vi "RoiSelectionCoordinatesAndorNull_FGV.vi"(8 "error in":errorcluster, 10 "FGV_Control":enum16{"Set", "Get"}(ring), 11 "ROI Coordinates in":T1) -> (0 "error out":errorcluster, 3 "ROI Coordinates out":T1)   [LabVIEW 2010]
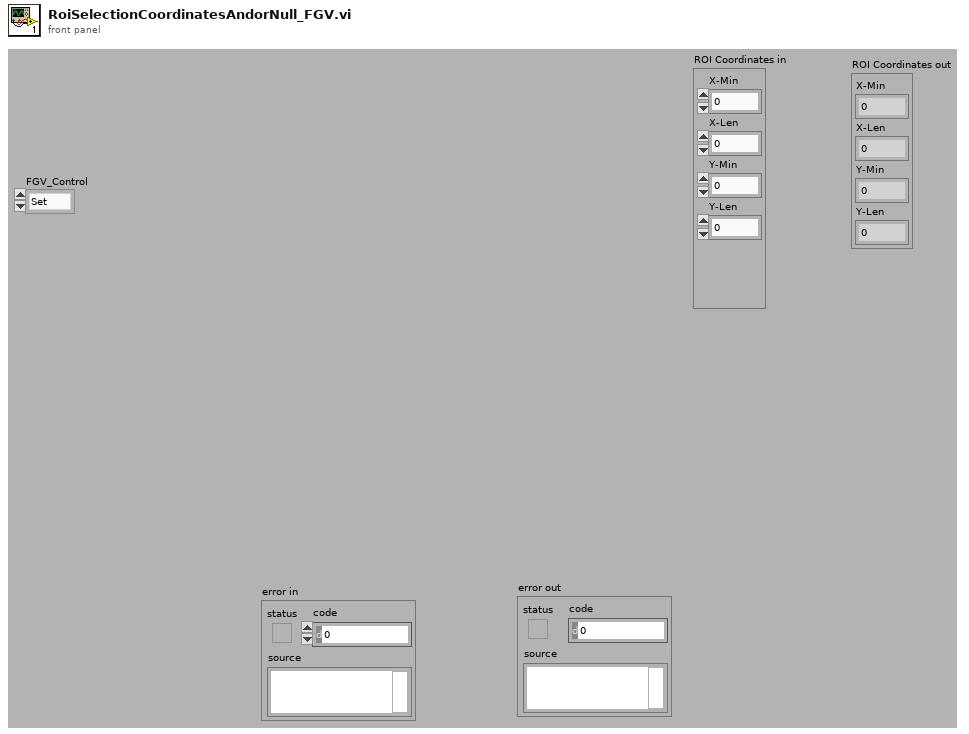
[diagram p1: front panel]
types:
  T1 = cluster{"X-Min":i32, "X-Len":i32, "Y-Min":i32, "Y-Len":i32}
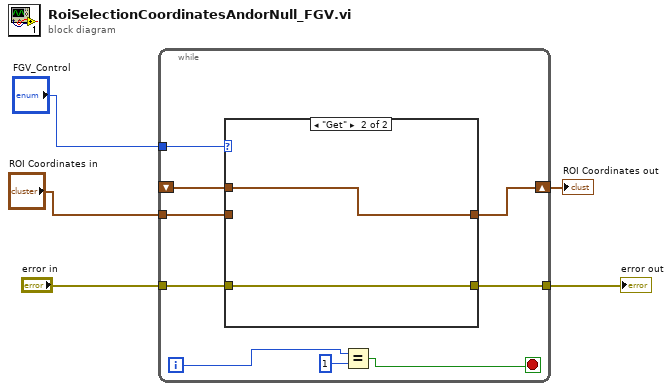
[diagram p0: block diagram]
diagram:
  n1 = while {
    tunnel: "FGV_Control" -> [w14]
    tunnel: "ROI Coordinates in" -> [w13]
    shift-right: [w12] -> w2
    shift-left: _ -> [w11]
    tunnel: "error in" -> [w7]
    tunnel: [w6] -> w4
    i -> [w8]
    stop <- w9 stop-if-true
    n2 = case shown="\"Get\"" w14 {
      tunnel: w13 -> [w16 _]
      tunnel: [w16 w18] -> w12
      tunnel: w11 -> [_ w18]
      tunnel: w7 -> [w15 w17]
      tunnel: [w15 w17] -> w6
      frame "Set", Default {
      }
      frame "Get" {
      }
    }
    n3 = Equal?(x=w8, y=1) -> (x = y?=w9:bool)
  }
  "error out" <- w4
  "ROI Coordinates out" <- w2
